vi "SetMovingVelocity.vi"(8 "error in (no error)":errorcluster, 11 "Tapedrive_ESP301 in":refnum<class "Tapedrive_ESP301.lvclass">) -> (0 "error out":errorcluster, 3 "Tapedrive_ESP301 out":refnum<class "Tapedrive_ESP301.lvclass">)   [LabVIEW 2013, in "Tapedrive_ESP301.lvclass"]
uses:
  Tapedrive_ESP301.lvclass
panel:
  out "Array 2":dbl[](array[numeric])
  out "Array":bool[](array[boolean])
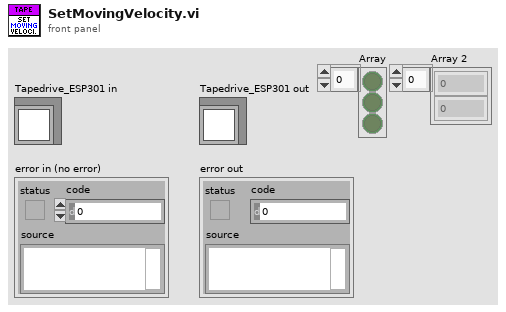
[diagram p1: front panel]
types:
  T1 = cluster{"Axis 1":cluster{"Value":dbl, "Min":dbl, "Max":dbl, "StepSize":dbl, "Tolerance":dbl, "ValueActual":dbl}, "Axis 2":cluster{"Value":dbl, "Min":dbl, "Max":dbl, "StepSize":dbl, "Tolerance":dbl, "ValueActual":dbl}}
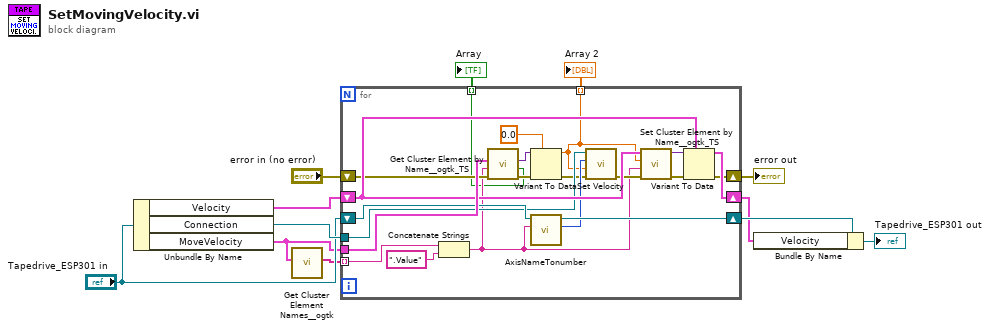
[diagram p0: block diagram]
diagram:
  n1 = Unbundle By Name("Tapedrive_ESP301 in") -> ("Velocity"=w12:T1, "Connection"=w7:refnum<visa-resource-name>, "MoveVelocity"=w4:T1)
  n2 = call <userlib>:"Get Cluster Element Names__ogtk.vi"("Cluster"=w4) -> ("Element Names"=w3:string[])  [unwired: 9 in, 1 out]
  n3 = for {
    tunnel: w3 -> [w16] mode=indexing
    tunnel: w4 -> [w32]
    shift-right: [w26] -> w5
    shift-left: w12 -> [w27]
    shift-right: [w24] -> w10
    shift-left: "Tapedrive_ESP301 in" -> [w25]
    tunnel: w7 -> [w22]
    shift-right: [w18] -> w9
    shift-left: "error in (no error)" -> [w17]
    tunnel: [w14] -> w2 mode=indexing
    tunnel: [w13] -> w1 mode=indexing
    n4 = Concatenate Strings(w16, ".Value" ("string")) -> (w15:string)
    n5 = call "Get Cluster Element by Name__ogtk_TS.vi"("error in (no error)"=w17, "Element Name"=w15, "Cluster"=w32) -> ("error out"=w21:errorcluster, "found?"=w14:bool, "VElement"=w31:variant)  [unwired: 6 in]
    n6 = Variant To Data(error in=w21, type=0.0, Variant=w31) -> (data=w13:dbl, error out=w20:errorcluster)
    n7 = call "AxisNameTonumber.vi"("Channel"=w15, "Tapedrive_ESP301 in"=w25) -> ("Axis No."=w23:i16, "Tapedrive_ESP301 out"=w24:refnum<class "Tapedrive_ESP301.lvclass">)  [unwired: 8 in]
    n8 = call <instrlib>:"Set Velocity.vi"("error in (no error)"=w20, "Velocity (units/s)"=w13, "Axis (1)"=w23, "VISA resource name"=w22) -> ("error out"=w19:errorcluster)  [unwired: 2 in, 1 out]
    n9 = call "Set Cluster Element by Name__ogtk_TS.vi"("error in (no error)"=w19, "Element Name (\"\": New Element Data Name)"=w15, "New Element Value"=w13, "Cluster"=w27) -> ("error out"=w29:errorcluster, "VCluster out"=w28:variant)  [unwired: 5 in, 1 out]
    n10 = Variant To Data(error in=w29, type=w27, Variant=w28) -> (data=w26:T1, error out=w18:errorcluster)
  }
  "error out" <- w9
  "Array" <- w2
  "Array 2" <- w1
  n11 = Bundle By Name(cluster=w10, "Velocity"=w5) -> (→"Tapedrive_ESP301 out":refnum<class "Tapedrive_ESP301.lvclass">)
